vi "set initial CompareSettings.vi"(8 "error in":errorcluster, 10 "Project Name":string="vicompare.lvproj", 11 "Build Spec Name":string="1_diffmain") -> (0 "error out":errorcluster)   [LabVIEW 2016]
uses:
  controls/CL Args.ctl
  <vilib>/Utility/config.llb/Write Key (Boolean).vi
  <vilib>/Utility/config.llb/NI_LVConfig.lvlib
panel:
  in  "settings":T1={"-noattr"=TRUE, "-nofp"=TRUE, "-nofppos"=TRUE, "-nobd"=FALSE, "-nobdcosm"=TRUE, "-nobdpos"=TRUE}
  in  "Manual":bool=TRUE caption="Utilize Manual Dialog"
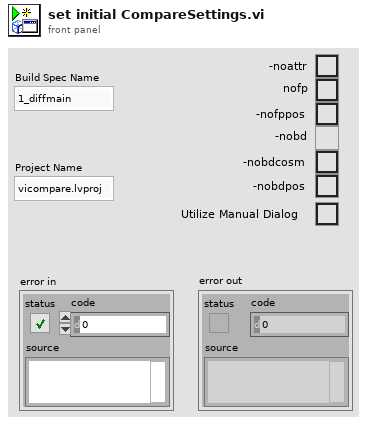
[diagram p1: front panel]
types:
  T1 = typedef "CL Args.ctl" = cluster{"-noattr":bool, "-nofp":bool, "-nofppos":bool, "-nobd":bool, "-nobdcosm":bool, "-nobdpos":bool}
  T2 = typedef "NI_LVConfig.lvlib/Config Data RefNum.ctl" = refnum<k1>
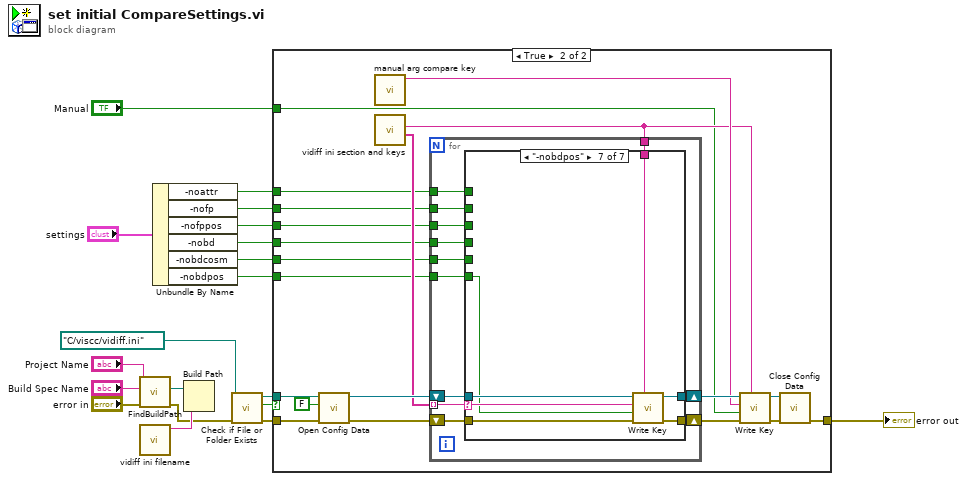
[diagram p0: block diagram]
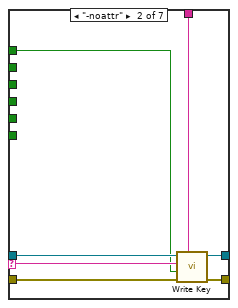
[diagram p4: hidden frame]
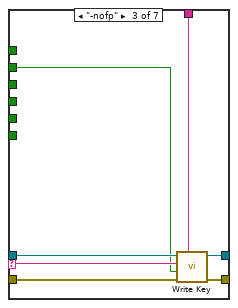
[diagram p5: hidden frame]
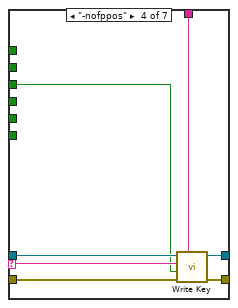
[diagram p6: hidden frame]
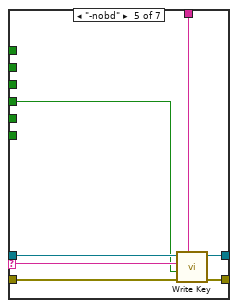
[diagram p7: hidden frame]
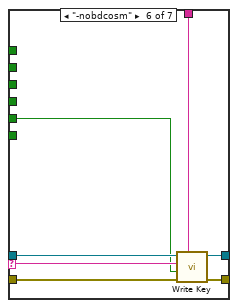
[diagram p8: hidden frame]
diagram:
  n1 = call "FindBuildPath.vi"("error in"="error in", "Build Spec Name"="Build Spec Name", "Project Name"="Project Name") -> ("error out"=w10:errorcluster, "Destination Path"=w15:path)  [unwired: 7 in]
  n2 = call "vidiff ini filename.vi"() -> ("VIdiff INI file"=w16:string)  [unwired: 11 in]
  n3 = Unbundle By Name("settings") -> ("-noattr"=w4:bool, "-nofp"=w5:bool, "-nofppos"=w3:bool, "-nobd"=w6:bool, "-nobdcosm"=w7:bool, "-nobdpos"=w2:bool)
  n4 = Build Path(base path=w15, name or relative path=w16) -> ()  [unwired: 1 out]
  n5 = call <vilib>:"Check if File or Folder Exists.vi"("error in (no error)"=w10, "path"=path "C:/viscc/vidiff.ini") -> ("error out"=w13:errorcluster, "file or folder exists?"=w12:bool, "dup path"=w14:path)  [unwired: 7 in]
  n6 = case shown="True" w12 {
    tunnel: w14 -> [_ w29]
    tunnel: [w20 w34] -> w17
    tunnel: w13 -> [w20 w30]
    tunnel: w6 -> [_ w27]
    tunnel: w5 -> [_ w26]
    tunnel: w7 -> [_ w25]
    tunnel: "Manual" -> [_ w24]
    tunnel: w4 -> [_ w23]
    tunnel: w3 -> [_ w22]
    tunnel: w2 -> [_ w21]
    frame False {
    }
    frame True {
      n7 = call <vilib>:"Open Config Data.vi"("error in (no error)"=w30, "create file if necessary (T)"=FALSE, "configuration file path"=w29) -> ("error out"=w39:errorcluster, "refnum"=w40:T2)  [unwired: 6 in, 1 out]
      n8 = call "manual arg compare key.vi"() -> ("manual key"=w33:string)  [unwired: 11 in]
      n9 = call "vidiff ini section and keys.vi"() -> ("DiffArgKeyNames"=w31:string[], "Section"=w32:string)  [unwired: 10 in]
      n10 = for {
        tunnel: w32 -> [w48]
        shift-right: [w50] -> w38
        shift-left: w40 -> [w52]
        shift-right: [w49] -> w36
        shift-left: w39 -> [w51]
        tunnel: w31 -> [w47] mode=indexing
        tunnel: w27 -> [w46]
        tunnel: w26 -> [w45]
        tunnel: w23 -> [w44]
        tunnel: w25 -> [w43]
        tunnel: w22 -> [w42]
        tunnel: w21 -> [w41]
        n11 = case shown="\"-nobdpos\"" w47 {
          selector: w47 -> [_ w56 w63 w70 w77 w84 w91]
          tunnel: w52 -> [w54 w61 w68 w75 w82 w89 w96]
          tunnel: w51 -> [w53 w60 w67 w74 w81 w88 w95]
          tunnel: [w54 w59 w66 w73 w80 w87 w94] -> w50
          tunnel: [w53 w58 w65 w72 w79 w86 w93] -> w49
          tunnel: w48 -> [_ w57 w64 w71 w78 w85 w92]
          tunnel: w46 -> [_ _ _ _ w76 _ _]
          tunnel: w45 -> [_ _ w62 _ _ _ _]
          tunnel: w44 -> [_ w55 _ _ _ _ _]
          tunnel: w43 -> [_ _ _ _ _ w83 _]
          tunnel: w42 -> [_ _ _ w69 _ _ _]
          tunnel: w41 -> [_ _ _ _ _ _ w90]
          frame Default {
          }
          frame "-noattr" {
            n12 = call-poly <vilib>:"Write Key.vi"("section"=w57, "error in (no error)"=w60, "value"=w55, "key"=w56, "refnum"=w61) -> ("error out"=w58:errorcluster, "refnum out"=w59:T2)  [unwired: 4 in, 1 out]
          }
          frame "-nofp" {
            n13 = call-poly <vilib>:"Write Key.vi"("section"=w64, "error in (no error)"=w67, "value"=w62, "key"=w63, "refnum"=w68) -> ("error out"=w65:errorcluster, "refnum out"=w66:T2)  [unwired: 4 in, 1 out]
          }
          frame "-nofppos" {
            n14 = call-poly <vilib>:"Write Key.vi"("section"=w71, "error in (no error)"=w74, "value"=w69, "key"=w70, "refnum"=w75) -> ("error out"=w72:errorcluster, "refnum out"=w73:T2)  [unwired: 4 in, 1 out]
          }
          frame "-nobd" {
            n15 = call-poly <vilib>:"Write Key.vi"("section"=w78, "error in (no error)"=w81, "value"=w76, "key"=w77, "refnum"=w82) -> ("error out"=w79:errorcluster, "refnum out"=w80:T2)  [unwired: 4 in, 1 out]
          }
          frame "-nobdcosm" {
            n16 = call-poly <vilib>:"Write Key.vi"("section"=w85, "error in (no error)"=w88, "value"=w83, "key"=w84, "refnum"=w89) -> ("error out"=w86:errorcluster, "refnum out"=w87:T2)  [unwired: 4 in, 1 out]
          }
          frame "-nobdpos" {
            n17 = call-poly <vilib>:"Write Key.vi"("section"=w92, "error in (no error)"=w95, "value"=w90, "key"=w91, "refnum"=w96) -> ("error out"=w93:errorcluster, "refnum out"=w94:T2)  [unwired: 4 in, 1 out]
          }
        }
      }
      n18 = call-poly <vilib>:"Write Key.vi"("section"=w32, "error in (no error)"=w36, "value"=w24, "key"=w33, "refnum"=w38) -> ("error out"=w35:errorcluster, "refnum out"=w37:T2)  [unwired: 4 in, 1 out]
      n19 = call <vilib>:"Close Config Data.vi"("error in (no error)"=w35, "refnum"=w37) -> ("error out"=w34:errorcluster)  [unwired: 8 in, 1 out]
    }
  }
  "error out" <- w17
